vi "heap.vi"(11 "Service Request":refnum<class "Web Request.lvclass">) -> (0 "health_heart_rate":dbl, 1 "comment":string, 2 "psd":string, 3 "lf_hf":dbl, 4 "hf":dbl, 5 "lf":dbl, 6 "PN50":dbl, 7 "heart_rate":dbl, 8 "base_line_0":string, 9 "sdnn":string, 10 "org_graph":string)   [LabVIEW 2018]
uses:
  <vilib>/wsapi/Web Request.lvclass
  <vilib>/express/express analysis/Spectral/Block/exnSpectralBlock spectral measurements PSD poly.vi
  <vilib>/express/express analysis/Spectral/Block/exnSpectralBlock spectral measurements PSD WFM.vi
  <vilib>/express/express analysis/Spectral/XNode/ExpressSpectralMeasurementsBlockNode.xnode
  <vilib>/Analysis/NI_AALPro.lvlib
panel:
  out "integral of P(x)":dbl
  out "R-R interval(ms)":dbl[](array[numeric])
  out "SDNN(ms)":dbl[](array[numeric])
  out "R wave time":dbl[](array[numeric])
  out "Ninth_IMF":dbl[](graph)
  out "Eighth IMF":dbl[](graph)
  out "Seventh IMF":dbl[](graph)
  out "Sixth IMF":dbl[](graph)
  out "Fifth IMF":dbl[](graph)
  out "Fourth IMF":dbl[](graph)
  out "Third IMF":dbl[](graph)
  out "Second IMF":dbl[](graph)
  out "Num of IMF":i32
  out "First IMF":dbl[](graph)
  # "Use the Web Service Request input terminal to call the VIs on the Web Services palette. Do not remove it from the connector pane unless you don't need access to the palette."
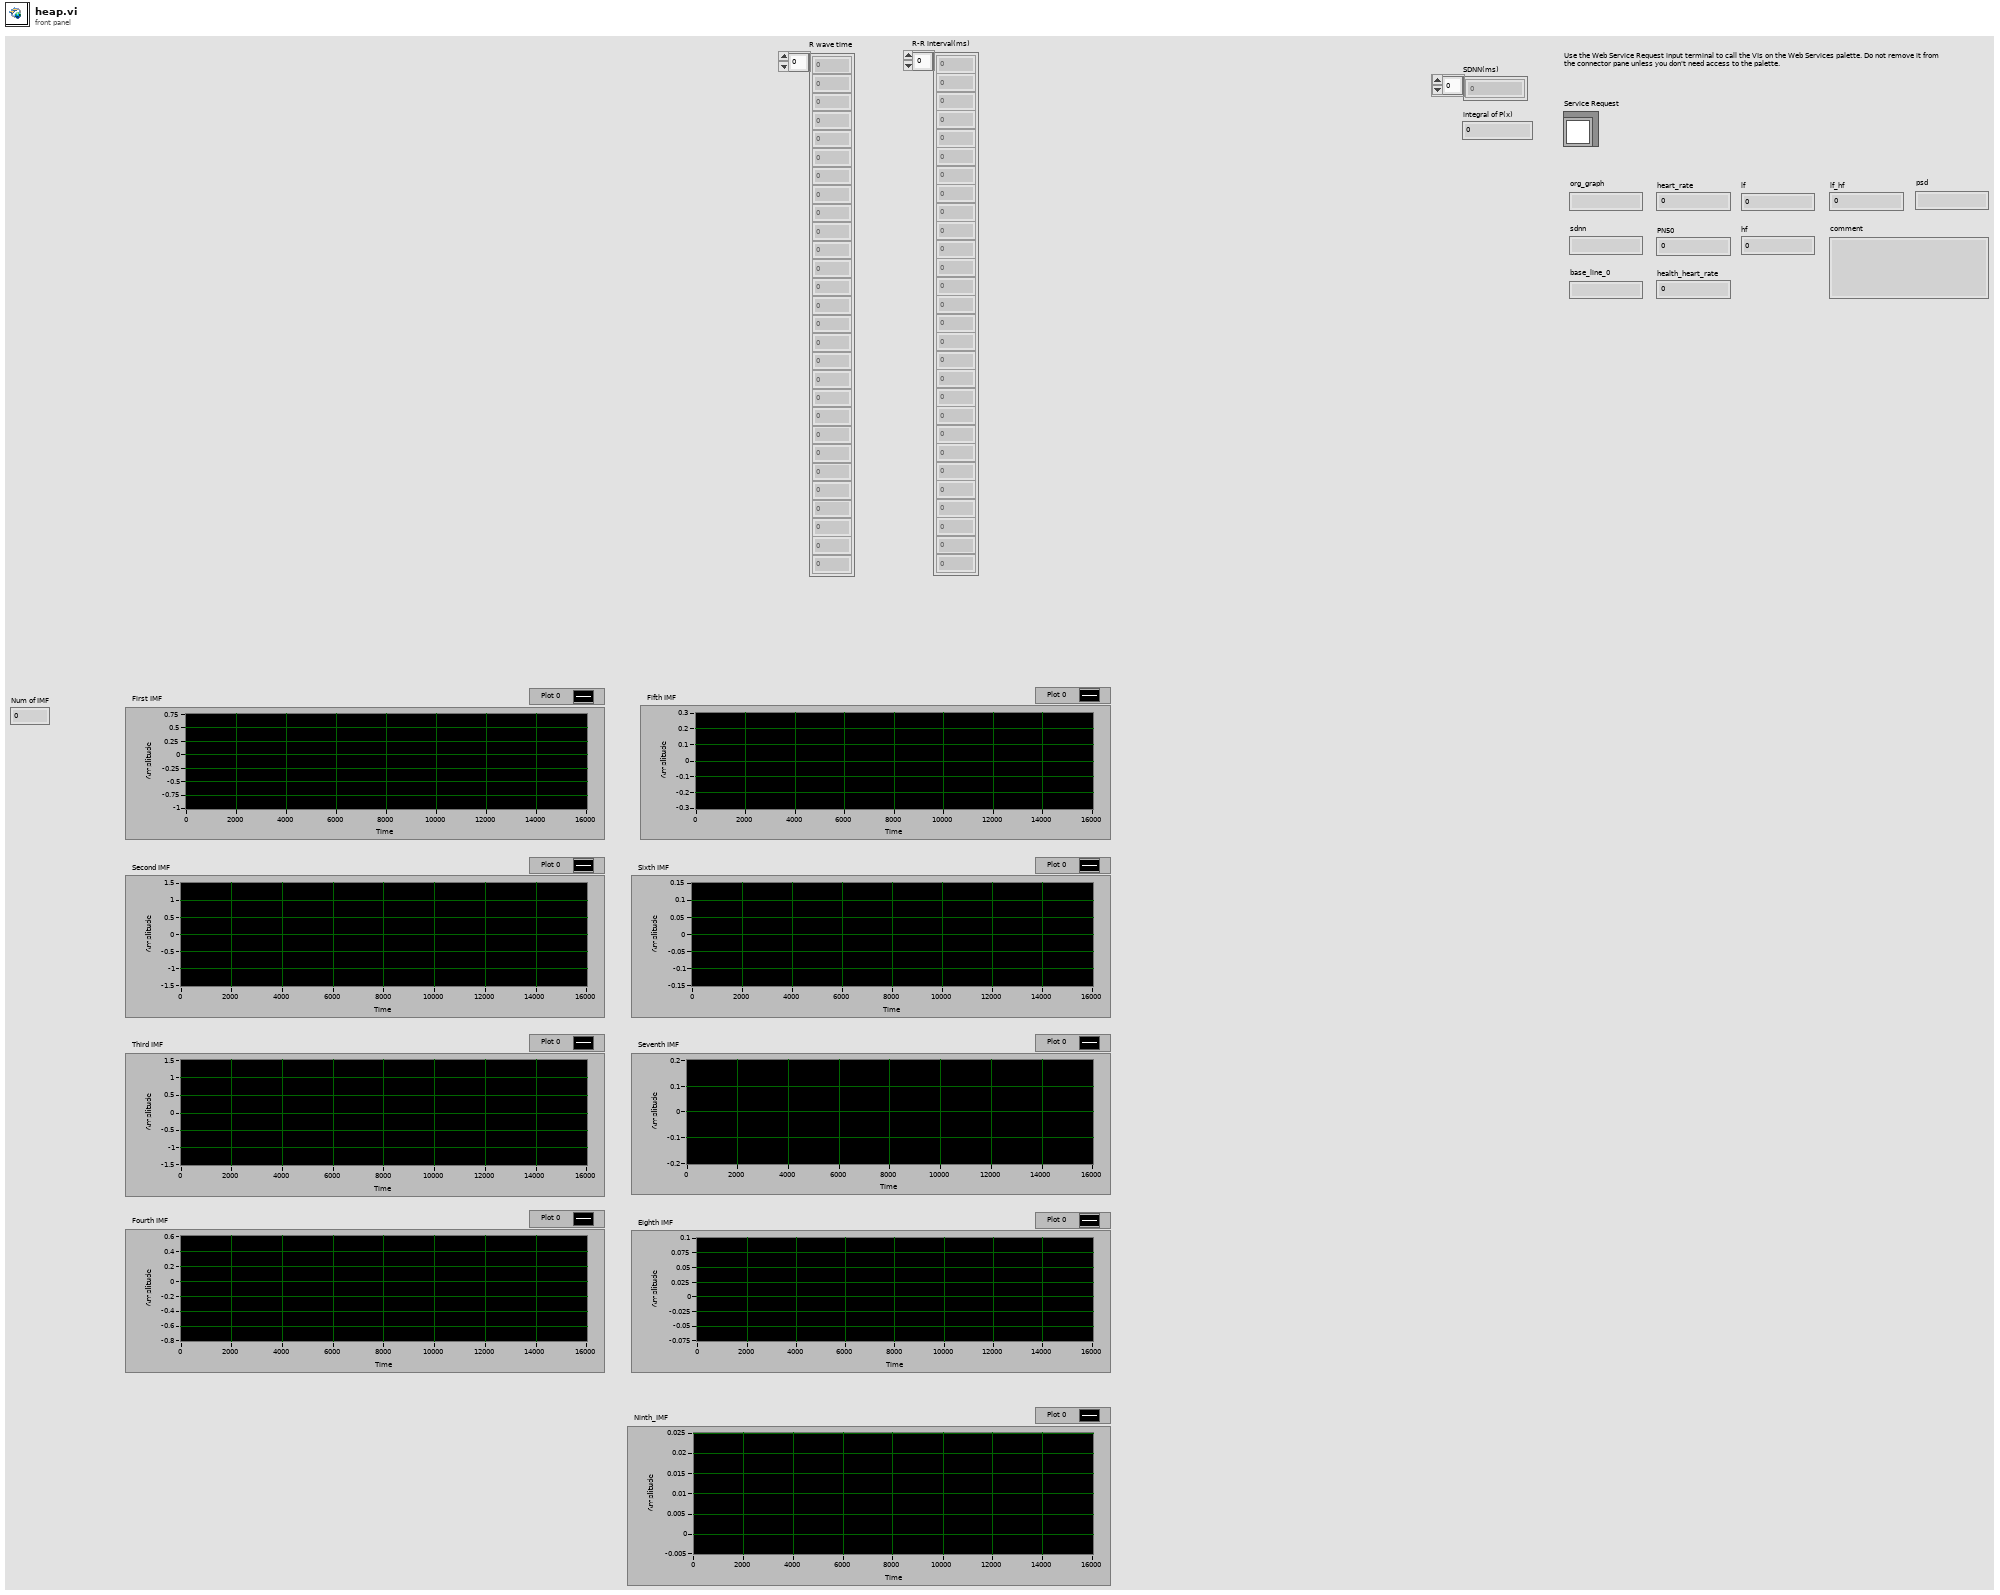
[diagram p1: front panel]
types:
  T1 = cluster{"averaging mode":u16, "weighting mode":u16, "number of averages":u32}
  T2 = cluster{"dB On (F)":bool, "unwrap phase (F)":bool, "convert to degree (F)":bool}
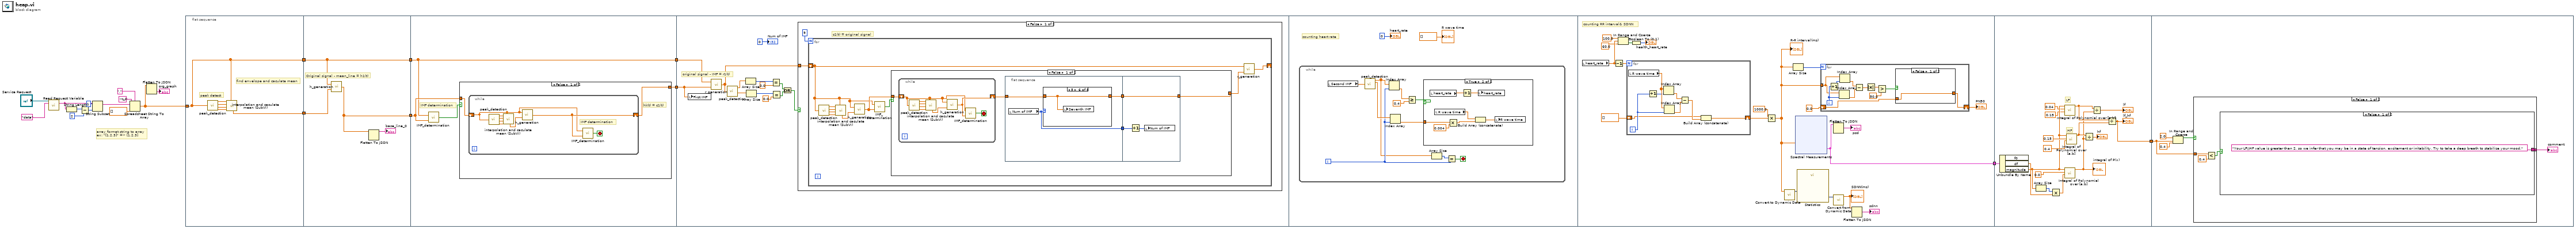
[diagram p0: block diagram]
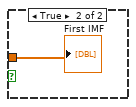
[diagram p2: hidden frame]
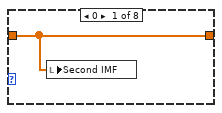
[diagram p3: hidden frame]
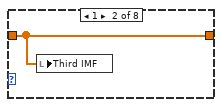
[diagram p4: hidden frame]
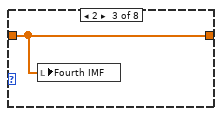
[diagram p5: hidden frame]
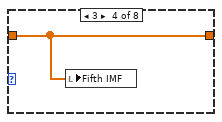
[diagram p6: hidden frame]
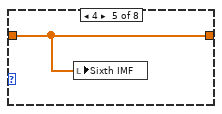
[diagram p7: hidden frame]
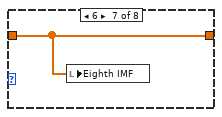
[diagram p8: hidden frame]
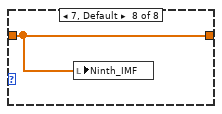
[diagram p9: hidden frame]
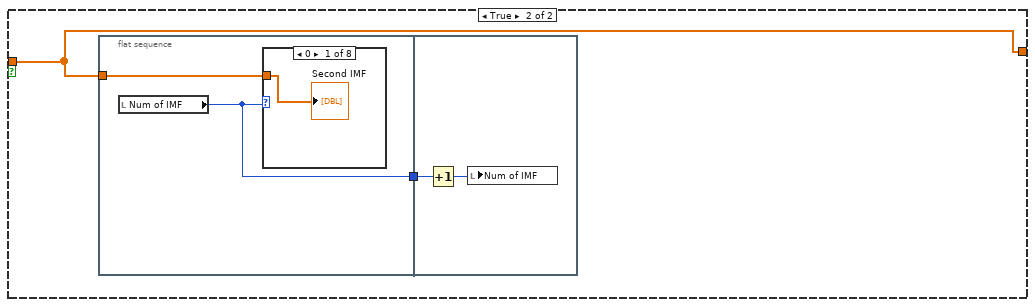
[diagram p10: hidden frame]
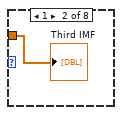
[diagram p11: hidden frame]
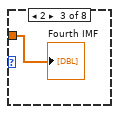
[diagram p12: hidden frame]
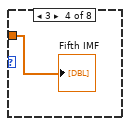
[diagram p13: hidden frame]
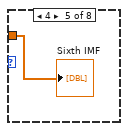
[diagram p14: hidden frame]
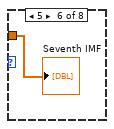
[diagram p15: hidden frame]
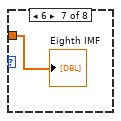
[diagram p16: hidden frame]
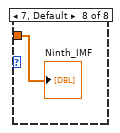
[diagram p17: hidden frame]
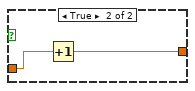
[diagram p20: hidden frame]
diagram:
  # "array format string to array\nex: \"[1,2,3]\" => [1,2,3]"
  n1 = call <vilib>:"Read Request Variable.vi"("LabVIEW Web Service Request"="Service Request", "variable name"="data") -> ("value"=w11:string)  [unwired: 11 in, 2 out]
  n2 = String Length(string=w11) -> (length=w17:i32)
  n3 = Subtract(x=w17, y=2) -> (x-y=w19:i32)
  n4 = String Subset(string=w11, offset (0)=1, length (rest)=w19) -> (substring=w15:string)
  n5 = Spreadsheet String To Array(delimiter (Tab)=",", format string="%f", spreadsheet string=w15, array type (2D Dbl)=dbl[] []) -> (array=w2:dbl[])
  n6 = Flatten To JSON(anything=w2) -> (JSON string=→"org_graph":string)  [unwired: 2 in, 1 out]
  n7 = flat-sequence {
    tunnel: w2 -> [w27]
    tunnel: [w27] -> w10
    tunnel: [w22] -> w9
    tunnel: w10 -> [w31]
    tunnel: [w28] -> w8
    tunnel: [w31] -> w7
    tunnel: w9 -> [w30]
    tunnel: w8 -> [w34]
    tunnel: [w32] -> w6
    tunnel: w7 -> [w32]
    tunnel: [w35] -> w5
    tunnel: w6 -> [w49]
    tunnel: w5 -> [w48]
    tunnel: [w137] -> w4
    tunnel: w4 -> [w197]
    tunnel: [w187] -> w3
    tunnel: w3 -> [w198]
    frame #0 {
      # "peak detect"
      # "find envelope and caculate mean"
      n8 = call "peak_detection.vi"("Array"=w27) -> ("upper"=w26:dbl[], "upper time"=w25:dbl[], "lower"=w24:dbl[], "lower time"=w23:dbl[])
      n9 = call "interpolation and caculate mean (SubVI).vi"("upper"=w26, "upper time"=w25, "lower"=w24, "lower time"=w23, "original"=w27) -> ("mean after interpolation"=w22:dbl[])  [unwired: 5 out]
    }
    frame #1 {
      # "Original signal - mean_line = h1(t)"
      n10 = call "h_generation.vi"("every_mean_points"=w30, "Y"=w31) -> ("h(t)"=w28:dbl[])
      n11 = Flatten To JSON(anything=w28) -> (JSON string=→"base_line_0":string)  [unwired: 2 in, 1 out]
    }
    frame #2 {
      # "IMF determination"
      n12 = call "IMF_determination.vi"("h(t)"=w34, "original signal"=w32) -> ("x .and. y?"=w33:bool)
      n13 = case shown="False" w33 {
        tunnel: w34 -> [w37 w46]
        tunnel: [w36 _] -> w35
        frame False {
          # "hk(t) = c1(t)"
          n14 = while {
            shift-right: [w40] -> w36
            shift-left: w37 -> [w38]
            stop <- w39 stop-if-true
            # "IMF determination"
            n15 = call "peak_detection.vi"("Array"=w38) -> ("upper"=w45:dbl[], "upper time"=w44:dbl[], "lower"=w43:dbl[], "lower time"=w42:dbl[])
            n16 = call "interpolation and caculate mean (SubVI).vi"("upper"=w45, "upper time"=w44, "lower"=w43, "lower time"=w42, "original"=w38) -> ("mean after interpolation"=w41:dbl[])  [unwired: 5 out]
            n17 = call "h_generation.vi"("every_mean_points"=w41, "Y"=w38) -> ("h(t)"=w40:dbl[])
            n18 = call "IMF_determination.vi"("h(t)"=w40, "original signal"=w38) -> ("x .and. y?"=w39:bool)
          }
        }
        frame True {
          "First IMF" <- w46
        }
      }
    }
    frame #3 {
      # "original signal - IMF = r1(t)"
      n19 = local write "First IMF"(w48) -> ()
      n20 = call "r_generation.vi"("IMF_points"=w48, "Original_signal"=w49) -> ("r1(t)"=w54:dbl[])
      n21 = call "peak_detection.vi"("Array"=w54) -> ("upper"=w53:dbl[], "lower"=w51:dbl[])  [unwired: 2 out]
      n22 = Array Size(array=w53) -> (size(s)=w52:i32)
      n23 = Array Size(array=w51) -> (size(s)=w50:i32)
      n24 = Equal?(x=w52, y=0.0) -> (x = y?=w57:bool)
      n25 = Equal?(x=w50, y=0.0) -> (x = y?=w56:bool)
      n26 = Or(x=w57, y=w56) -> (x .or. y?=w55:bool)
      n27 = case shown="False" w55 {
        tunnel: w54 -> [w61 _]
        frame False {
          # "c1(t) = original signal"
          n28 = for {
            N: 9 -> [_]
            shift-right: [w62] -> _
            shift-left: w61 -> [w64]
            n29 = call "peak_detection.vi"("Array"=w64) -> ("upper"=w71:dbl[], "upper time"=w70:dbl[], "lower"=w69:dbl[], "lower time"=w68:dbl[])
            n30 = call "interpolation and caculate mean (SubVI).vi"("upper"=w71, "upper time"=w70, "lower"=w69, "lower time"=w68, "original"=w64) -> ("mean after interpolation"=w67:dbl[])  [unwired: 5 out]
            n31 = call "h_generation.vi"("every_mean_points"=w67, "Y"=w64) -> ("h(t)"=w66:dbl[])
            n32 = call "IMF_determination.vi"("h(t)"=w66, "original signal"=w64) -> ("x .and. y?"=w65:bool)
            n33 = case shown="False" w65 {
              tunnel: w66 -> [w76 w99]
              tunnel: [w74 w99] -> w63
              frame False {
                n34 = while {
                  shift-right: [w92] -> w75
                  shift-left: w76 -> [w91]
                  stop <- w93 stop-if-true
                  n35 = call "peak_detection.vi"("Array"=w91) -> ("upper"=w98:dbl[], "upper time"=w97:dbl[], "lower"=w96:dbl[], "lower time"=w95:dbl[])
                  n36 = call "interpolation and caculate mean (SubVI).vi"("upper"=w98, "upper time"=w97, "lower"=w96, "lower time"=w95, "original"=w91) -> ("mean after interpolation"=w94:dbl[])  [unwired: 5 out]
                  n37 = call "h_generation.vi"("every_mean_points"=w94, "Y"=w91) -> ("h(t)"=w92:dbl[])
                  n38 = call "IMF_determination.vi"("h(t)"=w92, "original signal"=w91) -> ("x .and. y?"=w93:bool)
                }
                n39 = flat-sequence {
                  tunnel: w75 -> [w79]
                  tunnel: [w78] -> w73
                  tunnel: [w77] -> w72
                  tunnel: [w90] -> w74
                  tunnel: w73 -> [w90]
                  tunnel: w72 -> [w89]
                  frame #0 {
                    n40 = local read "Num of IMF"() -> (w77:i32)
                    n41 = case shown="5" w77 {
                      tunnel: w79 -> [w80 w81 w82 w83 w84 w85 w86 w87]
                      tunnel: [w80 w81 w82 w83 w84 w85 w86 w87] -> w78
                      frame 0 {
                        n42 = local write "Second IMF"(w80) -> ()
                      }
                      frame 1 {
                        n43 = local write "Third IMF"(w81) -> ()
                      }
                      frame 2 {
                        n44 = local write "Fourth IMF"(w82) -> ()
                      }
                      frame 3 {
                        n45 = local write "Fifth IMF"(w83) -> ()
                      }
                      frame 4 {
                        n46 = local write "Sixth IMF"(w84) -> ()
                      }
                      frame 5 {
                        n47 = local write "Seventh IMF"(w85) -> ()
                      }
                      frame 6 {
                        n48 = local write "Eighth IMF"(w86) -> ()
                      }
                      frame 7, Default {
                        n49 = local write "Ninth_IMF"(w87) -> ()
                      }
                    }
                  }
                  frame #1 {
                    n50 = Increment(x=w89) -> (x+1=w88:i32)
                    n51 = local write "Num of IMF"(w88) -> ()
                  }
                }
              }
              frame True {
                n52 = flat-sequence {
                  tunnel: w99 -> [w102]
                  tunnel: [w101] -> w100
                  tunnel: w100 -> [w112]
                  frame #0 {
                    n53 = local read "Num of IMF"() -> (w101:i32)
                    n54 = case shown="0" w101 {
                      tunnel: w102 -> [w103 w104 w105 w106 w107 w108 w109 w110]
                      frame 0 {
                        "Second IMF" <- w103
                      }
                      frame 1 {
                        "Third IMF" <- w104
                      }
                      frame 2 {
                        "Fourth IMF" <- w105
                      }
                      frame 3 {
                        "Fifth IMF" <- w106
                      }
                      frame 4 {
                        "Sixth IMF" <- w107
                      }
                      frame 5 {
                        "Seventh IMF" <- w108
                      }
                      frame 6 {
                        "Eighth IMF" <- w109
                      }
                      frame 7, Default {
                        "Ninth_IMF" <- w110
                      }
                    }
                  }
                  frame #1 {
                    n55 = Increment(x=w112) -> (x+1=w111:i32)
                    n56 = local write "Num of IMF"(w111) -> ()
                  }
                }
              }
            }
            n57 = call "r_generation.vi"("IMF_points"=w63, "Original_signal"=w64) -> ("r1(t)"=w62:dbl[])
          }
        }
        frame True {
        }
      }
      "Num of IMF" <- 0
    }
    frame #4 {
      # "counting heart rate"
      n58 = while {
        i -> [w118]
        stop <- w123 stop-if-true
        n59 = local read "Second IMF"() -> (w115:dbl[])
        n60 = call "peak_detection.vi"("Array"=w115) -> ("upper"=w116:dbl[], "upper time"=w119:dbl[])  [unwired: 2 out]
        n61 = Index Array(array=w116, index=w118) -> (element=w122:dbl)
        n62 = Index Array(array=w119, index=w118) -> (element=w117:dbl)
        n63 = Greater Or Equal?(x=w122, y=0.4) -> (x >= y?=w120:bool)
        n64 = case shown="True" w120 {
          tunnel: w117 -> [_ w129]
          frame False {
          }
          frame True {
            n65 = local read "heart_rate"() -> (w130:dbl)
            n66 = local read "R wave time"() -> (w126:dbl[])
            n67 = Multiply(x=w129, y=0.004) -> (x*y=w127:dbl)
            n68 = Increment(x=w130) -> (x+1=w131:dbl)
            n69 = Build Array (concatenate)(w126, w127) -> (w125:dbl[])
            n70 = local write "heart_rate"(w131) -> ()
            n71 = local write "R wave time"(w125) -> ()
          }
        }
        n72 = Array Size(array=w116) -> (size(s)=w124:i32)
        n73 = Equal?(x=w124, y=w118) -> (x = y?=w123:bool)
      }
      "heart_rate" <- 0
      "R wave time" <- dbl[] []
    }
    frame #5 {
      # "counting RR interval& SDNN"
      n74 = local read "heart_rate"() -> (w136:dbl)
      n75 = Decrement(x=w136) -> (x-1=w149:dbl)
      n76 = In Range and Coerce(upper limit=100.0, x=w136, lower limit=60.0) -> (In Range?=w133:bool)  [unwired: 1 out]
      n77 = for {
        N: w149 -> [_]
        shift-right: [w174] -> w145
        shift-left: dbl[] [] -> [w175]
        i -> [w177]
        n78 = local read "R wave time"() -> (w181:dbl[])
        n79 = Increment(x=w177) -> (x+1=w180:i32)
        n80 = Index Array(array=w181, index=w180) -> (element=w179:dbl)
        n81 = Index Array(array=w181, index=w177) -> (element=w178:dbl)
        n82 = Subtract(x=w179, y=w178) -> (x-y=w176:dbl)
        n83 = Build Array (concatenate)(w175, w176) -> (w174:dbl[])
      }
      n84 = Boolean To (0,1)(Boolean=w133) -> (0, 1=→"health_heart_rate":i16)
      n85 = Multiply(x=1000.0, y=w145) -> (x*y=w141:dbl[])
      "R-R interval(ms)" <- w141
      n86 = call "Convert to Dynamic Data"("Array"=w141) -> ("Dynamic Data Type"=w148:dynamicdata)  [unwired: 3 in]
      n87 = Array Size(array=w141) -> (size(s)=w144:i32)
      n88 = xnode "Spectral Measurements"("Signals"=w141) -> ("PSD"=w137:cluster{"f0":dbl, "df":dbl, "magnitude":dbl[]})  [unwired: 1 in, 1 out]
      n89 = call "Statistics"("Signals"=w148) -> ("Standard Dev"=w147:dynamicdata)  [unwired: 25 in, 1 out]
      n90 = for {
        N: w144 -> [_]
        tunnel: w141 -> [w159]
        shift-right: [w151] -> w143
        shift-left: 0.0 -> [w152]
        i -> [w160]
        n91 = Increment(x=w160) -> (x+1=w161:i32)
        n92 = Index Array(array=w159, index=w160) -> (element=w158:dbl)
        n93 = Index Array(array=w159, index=w161) -> (element=w157:dbl)
        n94 = Subtract(x=w157, y=w158) -> (x-y=w156:dbl)
        n95 = Absolute Value(x=w156) -> (abs(x)=w155:dbl)
        n96 = Greater?(x=w155, y=50.0) -> (0:w153:bool)
        n97 = case shown="False" w153 {
          tunnel: w152 -> [w162 w164]
          tunnel: [w162 w163] -> w151
          frame False {
          }
          frame True {
            n98 = Increment(x=w164) -> (x+1=w163:dbl)
          }
        }
      }
      "PN50" <- w143
      n99 = Flatten To JSON(anything=w137) -> (JSON string=→"psd":string)  [unwired: 2 in, 1 out]
      n100 = call "Convert from Dynamic Data"("Dynamic Data Type"=w147) -> ("Array"=w140:dbl[])  [unwired: 3 in]
      "SDNN(ms)" <- w140
      n101 = Flatten To JSON(anything=w140) -> (JSON string=→"sdnn":string)  [unwired: 2 in, 1 out]
    }
    frame #6 {
      # "LF"
      # "HF"
      n102 = Unbundle By Name(w197) -> ("df"=w193:dbl, "magnitude"=w190:dbl[])  [unwired: 1 out]
      n103 = Array Size(array=w190) -> (size(s)=w195:i32)
      n104 = Multiply(x=w195, y=w193) -> (x*y=w194:dbl)
      n105 = call <vilib>:"Integral of Polynomial over [a,b].vi"("b"=0.15, "a"=0.04, "P(x)"=w190) -> ("integral of P(x)"=w186:dbl)  [unwired: 7 in, 1 out]
      n106 = call <vilib>:"Integral of Polynomial over [a,b].vi"("b"=w194, "a"=0.0, "P(x)"=w190) -> ("integral of P(x)"=w182:dbl)  [unwired: 7 in, 1 out]
      "integral of P(x)" <- w182
      n107 = call <vilib>:"Integral of Polynomial over [a,b].vi"("b"=0.4, "a"=0.15, "P(x)"=w190) -> ("integral of P(x)"=w184:dbl)  [unwired: 7 in, 1 out]
      n108 = Divide(x=w184, y=w182) -> (x/y=→"hf":dbl)
      n109 = Divide(x=w186, y=w182) -> (x/y=→"lf":dbl)
      n110 = Divide(x=w186, y=w184) -> (x/y=w187:dbl)
      "lf_hf" <- w187
    }
    frame #7 {
      n111 = In Range and Coerce(upper limit=2.0, x=w198, lower limit=0.4) -> (In Range?=w200:bool)  [unwired: 1 out]
      n112 = case shown="False" w200 {
        tunnel: [w203 "Your LF\\HL value is within the normal range. We assume that your mood is comfortable and stable. Please keep it up."] -> w199
        tunnel: w198 -> [w204 _]
        frame False {
          n113 = Less?(x=w204, y=0.4) -> (x < y?=w206:bool)
          n114 = case shown="False" w206 {
            tunnel: ["Your LF\\HF value is greater than 2, so we infer that you may be in a state of tension, excitement or irritability. Try to take a deep breath to stabilize your mood." "Your LF\\HF value is less than 0.4, so we speculate that you are in a state of depression. I suggest you go out for a walk to watch the scenery or chat with friends."] -> w203
            frame False {
            }
            frame True {
            }
          }
        }
        frame True {
        }
      }
      "comment" <- w199
    }
  }
